vi "Read Message from Image.vi"(7 "I_Mixed Coordinates":i32[][](array[numeric]), 8 "I_Sigma":i16, 9 "I_Number of columns":i16, 10 "I_Number of rows":i16, 11 "I_Image Data":T1) -> (2 "O_Text":i16[](array[numeric]), 3 "O_Image Data":T1)   [LabVIEW 2015]
uses:
  <vilib>/picture/picture.llb/imagedata.ctl
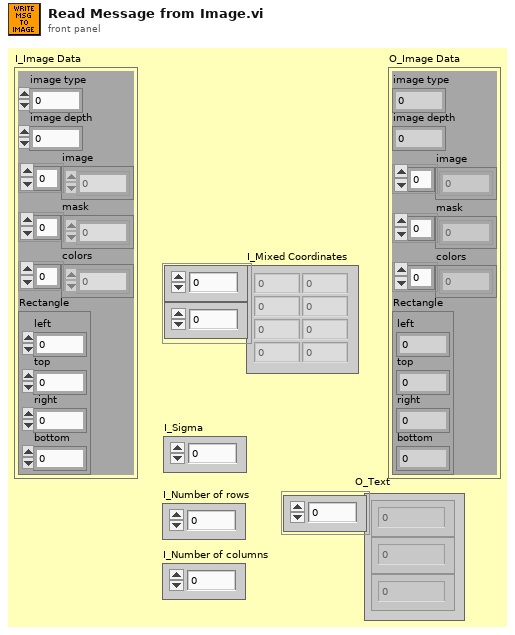
[diagram p1: front panel]
types:
  T1 = typedef "imagedata.ctl" = cluster{"image type":i32, "image depth":i32, "image":u8[], "mask":u8[], "colors":u32[], "Rectangle":cluster{"left":i16, "top":i16, "right":i16, "bottom":i16}}
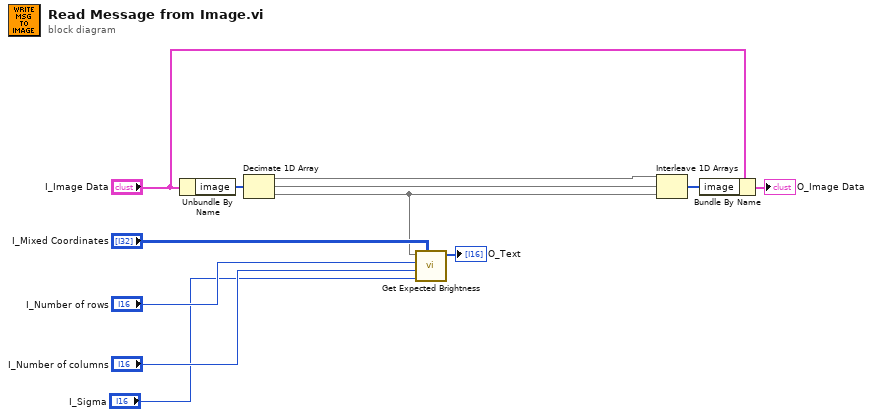
[diagram p0: block diagram]
diagram:
  n1 = Unbundle By Name("I_Image Data") -> ("image"=w12:u8[])
  n2 = Decimate 1D Array(w12) -> (w10:u8[], w11:u8[], w5:u8[])
  n3 = call "Get Expected Brightness.vi"("I_Mixed Coordinates"="I_Mixed Coordinates", "I_Sigma"="I_Sigma", "I_Number of columns"="I_Number of columns", "I_Number of rows"="I_Number of rows", "I_Blue Component"=w5) -> ("O_Text"=→"O_Text":i16[])  [unwired: 6 in]
  n4 = Interleave 1D Arrays(w10, w11, w5) -> (w9:u8[])
  n5 = Bundle By Name(cluster="I_Image Data", "image"=w9) -> (→"O_Image Data":T1)
